vi "Creator Alias.vi"(11 "Base Actor in":refnum<class "Base Actor.lvclass">) -> (2 "Creator Alias":string)   [LabVIEW 2021, in "jettl.lvlib" / "Actor.lvlib" / "Base Actor.lvclass"]
uses:
  Base Actor.lvclass
  Base Actor.lvclass/Base Actor.ctl
  Addresses Strategy/Addresses Strategy/Addresses Strategy.lvclass
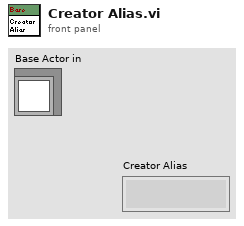
[diagram p1: front panel]
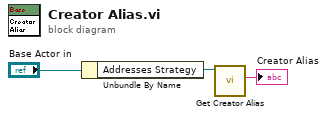
[diagram p0: block diagram]
diagram:
  n1 = Unbundle By Name("Base Actor in") -> ("Addresses Strategy"=w3:refnum<class "Addresses Strategy.lvclass">)
  n2 = call-dynamic "Get Creator Alias.vi"("Addresses Strategy in"=w3) -> ("Creator Alias"=→"Creator Alias":string)  [unwired: 10 in]
